vi "NewVSSNavigation.vi"() -> ()   [LabVIEW 2018]
uses:
  Vision_class/Old vision/SSL Detection Frame Simple Estimator Cameras VelCmd Folder/Core/AI Input.ctl
  Vision_class/Old vision/Controls/AI Robot.ctl
  Vision_class/Old vision/Controls/Functions Enum.ctl
  Vision_class/Old vision/Controls/AttackerStates.ctl
  Vision_class/Old vision/Controls/PathDests.ctl
  Vision_class/Old vision/Controls/PathDest.ctl
  VSSAttackerStates.ctl
  Vision_class/Old vision/SSL Detection Frame Simple Estimator Cameras VelCmd Folder/Core/AI Ball.ctl
  Vision_class/Old vision/SSL Detection Frame Simple Estimator Cameras VelCmd Folder/Core/Field Size.ctl
  Vision_class/Old vision/SSL Detection Frame Simple Estimator Cameras VelCmd Folder/Core/AI Judge.ctl
  Communication_class/Paths/MessageAI_State Folder/Intel/Command Enum.ctl
  Vision_class/Old vision/SSL Detection Frame Simple Estimator Cameras VelCmd Folder/Util/Events/Events.ctl
  Utilities_class/Utilities.lvclass
panel:
  in  "Penalty Shoot Out?":bool
  in  "PID gains Vel":T1={"proportional gain (Kc)"=0.6, "integral time (Ti, min)"=0.0, "derivative time (Td, min)"=0.0}
  in  "output angle":dbl
  in  "output xy":dbl
  in  "a1":dbl=10.0
  in  "a3":dbl=15.0
  in  "output inc":dbl
  in  "Test Mode":bool
  in  "VelNearBall":dbl=1.0 format="%#_13g"
  in  "Debug":bool
  in  "GoTo Navigation":bool
  in  "IA State Output in":T2
  out "IA State Output out":T2
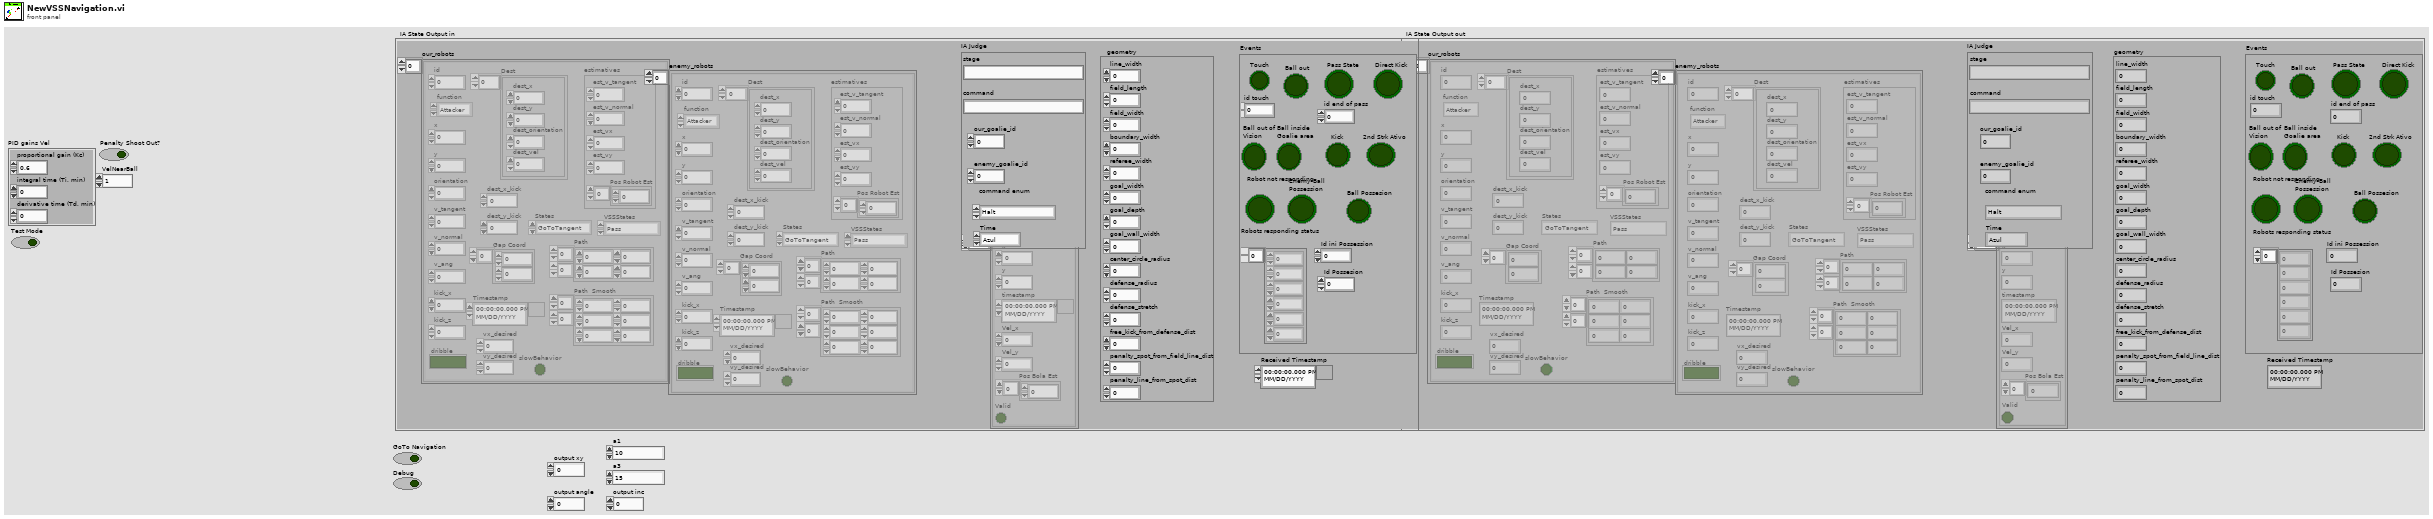
[diagram p1: front panel]
types:
  T1 = cluster{"proportional gain (Kc)":dbl, "integral time (Ti, min)":dbl, "derivative time (Td, min)":dbl}
  T2 = typedef "AI Input.ctl" = cluster{"our_robots":T3[], "enemy_robots":T3[], "balls":T9[], "geometry":T10, "IA Judge":T11, "Received Timestamp":timestamp, "Events":T13}
  T3 = typedef "AI Robot.ctl" = cluster{"id":u32, "function":T4, "x":dbl, "y":dbl, "orientation":dbl, "v_tangent":dbl, "v_normal":dbl, "v_ang":dbl, "kick_x":dbl, "kick_z":dbl, "dribble":bool, "Timestamp":timestamp, "estimatives":cluster{"est_v_tangent":dbl, "est_v_normal":dbl, "est_vx":dbl, "est_vy":dbl, "Pos Robot Est":dbl[]}, "dest_x_kick":dbl, "dest_y_kick":dbl, "Gap Coord":dbl[], "States":T5, "Path ":dbl[][], "Path  Smooth":dbl[][], "Dest":T6, "vx_desired":dbl, "vy_desired":dbl, "slowBehavior":bool, "VSSStates":T8}
  T4 = typedef "Functions Enum.ctl" = enum16{"2nd Striker", "Attacker", "Goalie", "Defender", "Striker", "Goto 0", "Dummy", "Kicker", "ZigZag 0", "ZigZag 1", "ZigZag 2", "ZigZag 3", "ZigZag 4", "ZigZag 5", "ZigZag 6", "ZigZag 7", "ZigZag 8", ""}
  T5 = typedef "AttackerStates.ctl" = enum16{"Pass", "GoToTangent", "BallGetting", "GoToKick", ""}
  T6 = typedef "PathDests.ctl" = T7[]
  T7 = typedef "PathDest.ctl" = cluster{"dest_x":dbl, "dest_y":dbl, "dest_orientation":dbl, "dest_vel":dbl}
  T8 = typedef "VSSAttackerStates.ctl" = enum16{"Pass", "GoToTangent", "BallGetting", "GoToKick", "Rotate anti-clockwise", "Rotate Clockwise", ""}
  T9 = typedef "AI Ball.ctl" = cluster{"x":dbl, "y":dbl, "timestamp":timestamp, "Vel_x":dbl, "Vel_y":dbl, "Pos Bola Est":dbl[], "Valid":bool}
  T10 = typedef "Field Size.ctl" = cluster{"line_width":u32, "field_length":u32, "field_width":u32, "boundary_width":u32, "referee_width":u32, "goal_width":u32, "goal_depth":u32, "goal_wall_width":u32, "center_circle_radius":u32, "defense_radius":u32, "defense_stretch":u32, "free_kick_from_defense_dist":u32, "penalty_spot_from_field_line_dist":u32, "penalty_line_from_spot_dist":u32}
  T11 = typedef "AI Judge.ctl" = cluster{"stage":string, "command":string, "our_goalie_id":dbl, "enemy_goalie_id":dbl, "command enum":T12, "Time":enum16{"Azul", "Amarelo"}}
  T12 = typedef "Command Enum.ctl" = enum16{"Halt", "Stop", "Force Start", "PKA Normal Start", "Prepare Kickoff Ally", "PKE Normal Start", "Prepare Kickoff Enemy", "Prepare Penalty Ally", "PPA Normal Start", "Prepare Penalty Enemy", "PPE Normal Start", "Direct Free Enemy", "Direct Free Ally", "Indirect Free Enemy", "Indirect Free Ally", "Timeout Enemy", "Timeout Ally", "Goal Enemy", "Goal Ally", "Ball Placement Enemy", "Ball Placement Ally", "Normal Half Time", "Extra Time Break", "Extra Half Time", "None", "Post Game"}
  T13 = typedef "Events.ctl" = cluster{"Touch":bool, "Ball out":bool, "id touch":dbl, "Ball out of \nVision":bool, "Ball inside \nGoalie area":bool, "Robot not responding":bool, "Robots responding status":dbl[], "Enemy Ball \nPossession":bool, "Pass State":bool, "id end of pass":dbl, "Kick":bool, "Id ini Possession":dbl, "Ball Possesion":bool, "Id Possesion":dbl, "Direct Kick":bool, "2nd Strk Ativo":bool}
  T14 = cluster{"est_v_tangent":dbl, "est_v_normal":dbl, "est_vx":dbl, "est_vy":dbl, "Pos Robot Est":dbl[]}
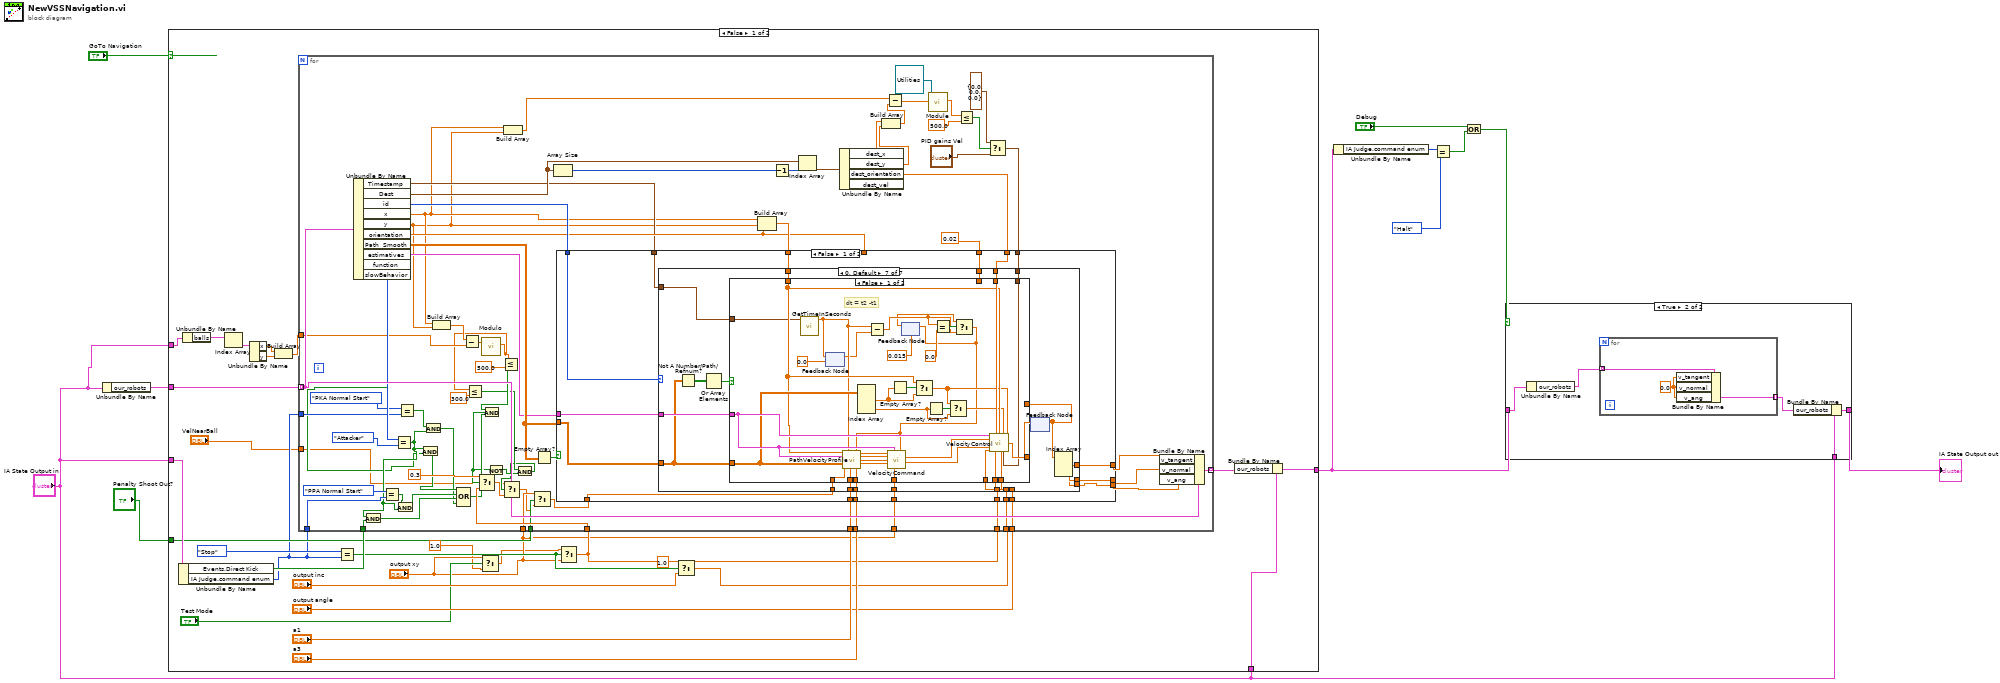
[diagram p0: block diagram]
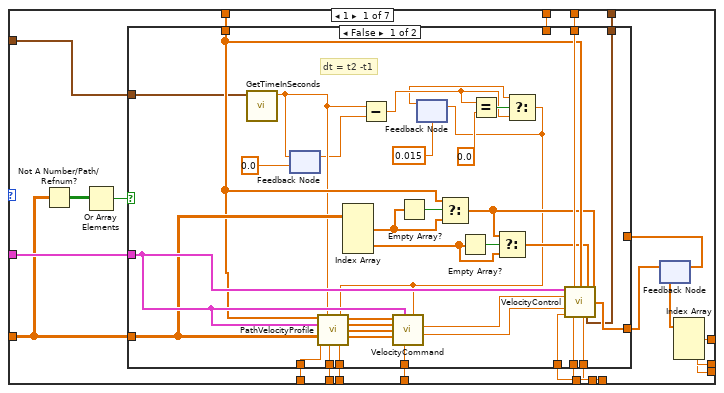
[diagram p2: hidden frame]
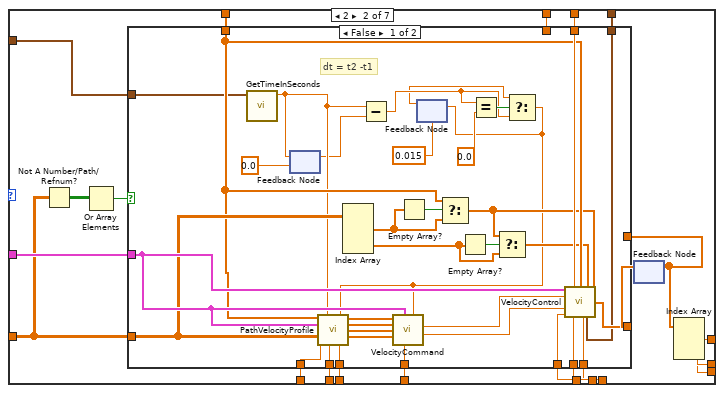
[diagram p4: hidden frame]
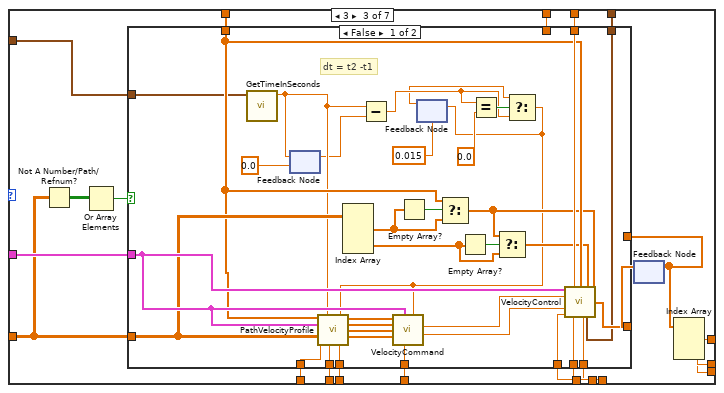
[diagram p6: hidden frame]
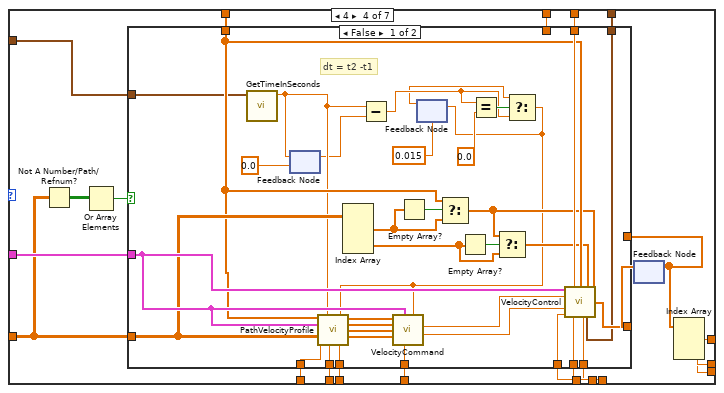
[diagram p8: hidden frame]
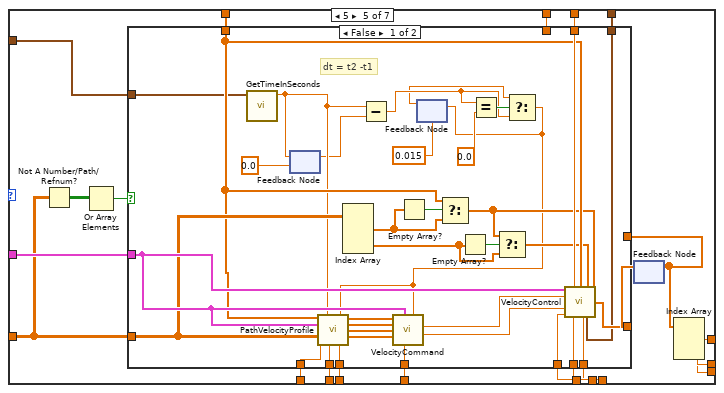
[diagram p10: hidden frame]
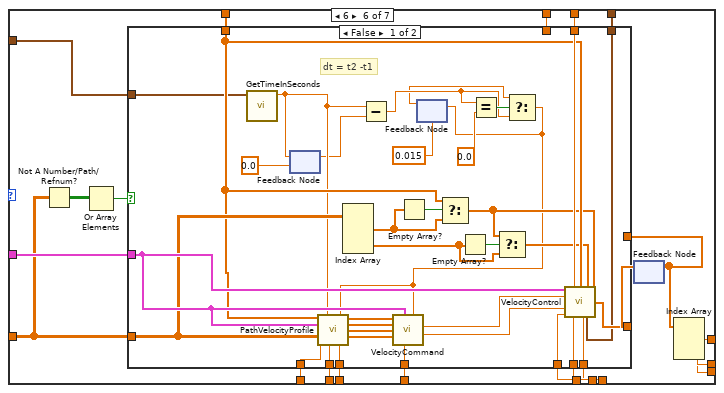
[diagram p12: hidden frame]
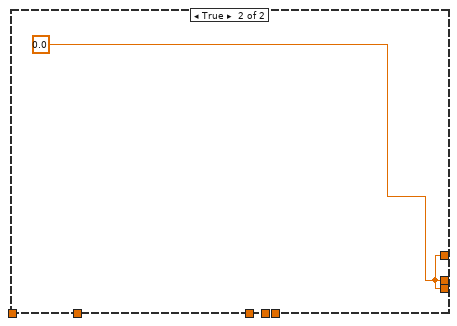
[diagram p15: hidden frame]
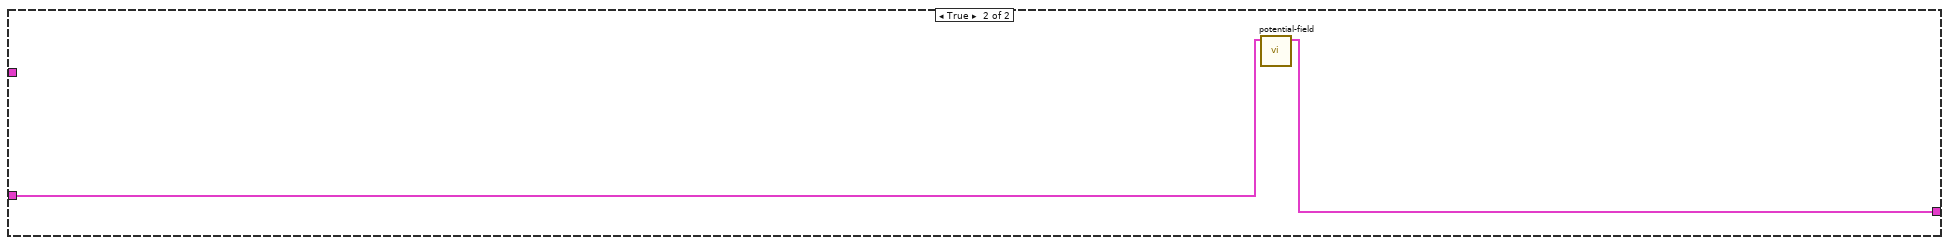
[diagram p16: hidden frame]
diagram:
  n1 = Unbundle By Name("IA State Output in") -> ("our_robots"=w11:T3[])
  n2 = case shown="False" "GoTo Navigation" {
    tunnel: w11 -> [w39 _]
    tunnel: [w36 w531] -> w8
    tunnel: "IA State Output in" -> [w32 w532]
    tunnel: "IA State Output in" -> [w37 _]
    tunnel: "IA State Output in" -> [w21 _]
    tunnel: "Penalty Shoot Out?" -> [w18 _]
    frame False {
      n3 = Unbundle By Name(w32) -> ("Events.Direct Kick"=w26:bool, "IA Judge.command enum"=w13:T12)
      n4 = Unbundle By Name(w21) -> ("balls"=w25:T9[])
      n5 = Index Array(array=w25) -> (element=w24:T9)  [unwired: 1 in]
      n6 = Unbundle By Name(w24) -> ("x"=w23:dbl, "y"=w22:dbl)
      n7 = Build Array(w23, w22) -> (w20:dbl[])
      n8 = Equal?(x=Command_Enum."Stop", y=w13) -> (x = y?=w19:bool)
      n9 = Select(t="output xy", s="Test Mode", f=1.0 ("t")) -> (s? t:f=w14:dbl)
      n10 = Select(t=w14, s=w19, f="output xy") -> (s? t:f=w30:dbl)
      n11 = Select(t=1.0, s=w19, f="output inc") -> (s? t:f=w28:dbl)
      n12 = for {
        tunnel: w39 -> [w112] mode=indexing
        tunnel: [w111] -> w38 mode=indexing
        tunnel: w30 -> [w89]
        tunnel: "a1" -> [w100]
        tunnel: "a3" -> [w99]
        tunnel: w28 -> [w95]
        tunnel: "output angle" -> [w94]
        tunnel: w30 -> [w93]
        tunnel: w13 -> [w87]
        tunnel: w26 -> [w81]
        tunnel: w13 -> [w79]
        tunnel: w20 -> [w70]
        tunnel: w18 -> [w67]
        tunnel: "output xy" -> [w66]
        tunnel: "output xy" -> [w51]
        tunnel: "VelNearBall" -> [w40]
        n13 = Unbundle By Name(w112) -> ("Timestamp"=w91:timestamp, "Dest"=w110:T6, "id"=w103:u32, "x"=w64:dbl, "y"=w63:dbl, "orientation"=w98:dbl, "Path  Smooth"=w104:dbl[][], "estimatives"=w101:T14, "function"=w80:T4, "slowBehavior"=w49:bool)
        n14 = Equal?(x=Command_Enum."PPA Normal Start", y=w87) -> (x = y?=w84:bool)
        n15 = Equal?(x=w80, y=Functions_Enum."Attacker") -> (x = y?=w76:bool)
        n16 = And(x=w76, y=w81) -> (x .and. y?=w82:bool)
        n17 = And(x=w84, y=w76) -> (x .and. y?=w83:bool)
        n18 = Equal?(x=Command_Enum."PKA Normal Start", y=w79) -> (x = y?=w77:bool)
        n19 = And(x=w76, y=w49) -> (x .and. y?=w85:bool)
        n20 = And(x=w77, y=w76) -> (x .and. y?=w75:bool)
        n21 = Build Array(w64, w63) -> (w71:dbl[])
        n22 = Compound Arithmetic op=OR(w85, w83, w82, w75) -> (w72:bool)
        n23 = Subtract(x=w71, y=w70) -> (x-y=w69:dbl[])
        n24 = call "Modulo.vi"("2D vector"=w69) -> ("Modulo"=w48:dbl)  [unwired: 10 in]
        n25 = Less Or Equal?(x=w48, y=300.0) -> (x <= y?=w46:bool)
        n26 = Less Or Equal?(x=w48, y=500.0) -> (x <= y?=w73:bool)
        n27 = And(x=w73, y=w72) -> (x .and. y?=w45:bool)
        n28 = Select(t=0.3, s=w45, f=w89) -> (s? t:f=w42:dbl)
        n29 = Not(x=w45) -> (.not. x?=w44:bool)
        n30 = Build Array(w64, w63) -> (w59:dbl[])
        n31 = And(x=w46, y=w44) -> (x .and. y?=w43:bool)
        n32 = Select(t=w40, s=w43, f=w42) -> (s? t:f=w41:dbl)
        n33 = Select(t=w66, s=w67, f=w41) -> (s? t:f=w65:dbl)
        n34 = Empty Array?(array=w104) -> (empty?=w105:bool)
        n35 = Array Size(array=w110) -> (size(s)=w109:i32)
        n36 = Build Array(w64, w63, w98) -> (w102:dbl[])
        n37 = Decrement(x=w109) -> (x-1=w108:i32)
        n38 = Index Array(array=w110, index=w108) -> (element=w107:T7)
        n39 = Unbundle By Name(w107) -> ("dest_x"=w62:dbl, "dest_y"=w61:dbl, "dest_orientation"=w106:dbl)  [unwired: 1 out]
        n40 = Build Array(w62, w61) -> (w60:dbl[])
        n41 = Subtract(x=w59, y=w60) -> (x-y=w58:dbl[])
        n42 = call-dynamic "Module.vi"("2D vector"=w58, "Utilities in"=refnum<class "Utilities.lvclass"> refnum) -> ("Modulo"=w56:dbl)  [unwired: 7 in, 2 out]
        n43 = Less Or Equal?(x=w56, y=500.0) -> (x <= y?=w54:bool)
        n44 = Select(t=T1 {"proportional gain (Kc)"=0.0, "integral time (Ti, min)"=0.0, "derivative time (Td, min)"=0.0}, s=w54, f="PID gains Vel") -> (s? t:f=w53:T1)
        n45 = case shown="False" w105 {
          tunnel: [w120 w530] -> w97
          tunnel: [w119 w530] -> w96
          tunnel: [w118 w530] -> w92
          tunnel: w103 -> [w116 _]
          tunnel: w104 -> [w122 _]
          tunnel: w106 -> [w123 _]
          tunnel: w102 -> [w121 _]
          tunnel: w101 -> [w124 _]
          tunnel: w65 -> [w130 _]
          tunnel: w100 -> [w129 _]
          tunnel: w99 -> [w128 _]
          tunnel: w98 -> [_ _]
          tunnel: w95 -> [w127 _]
          tunnel: w94 -> [w126 _]
          tunnel: w93 -> [w125 _]
          tunnel: w91 -> [w117 _]
          tunnel: 0.02 -> [w115 _]
          tunnel: w53 -> [w114 _]
          tunnel: w51 -> [w113 _]
          frame False {
            n46 = case shown="0, Default" w116 {
              tunnel: w130 -> [w151 w208 w265 w322 w379 w436 w493]
              tunnel: w129 -> [w150 w207 w264 w321 w378 w435 w492]
              tunnel: w128 -> [w149 w206 w263 w320 w377 w434 w491]
              tunnel: w127 -> [w148 w205 w262 w319 w376 w433 w490]
              tunnel: w126 -> [w147 w204 w261 w318 w375 w432 w489]
              tunnel: w125 -> [w146 w203 w260 w317 w374 w431 w488]
              tunnel: w124 -> [w145 w202 w259 w316 w373 w430 w487]
              tunnel: w123 -> [w144 w201 w258 w315 w372 w429 w486]
              tunnel: w122 -> [w136 w193 w250 w307 w364 w421 w478]
              tunnel: w121 -> [w143 w200 w257 w314 w371 w428 w485]
              tunnel: [w142 w199 w256 w313 w370 w427 w484] -> w120
              tunnel: [w141 w198 w255 w312 w369 w426 w483] -> w119
              tunnel: [w140 w197 w254 w311 w368 w425 w482] -> w118
              tunnel: w117 -> [w139 w196 w253 w310 w367 w424 w481]
              tunnel: w115 -> [w133 w190 w247 w304 w361 w418 w475]
              tunnel: w114 -> [w132 w189 w246 w303 w360 w417 w474]
              tunnel: w113 -> [w131 w188 w245 w302 w359 w416 w473]
              frame 1 {
                n47 = Not A Number/Path/Refnum?(number/path/refnum=w136) -> (NaN/Path/Refnum?=w135:bool[][])
                n48 = Or Array Elements(Boolean array=w135) -> (logical OR=w134:bool)
                n49 = feedback #1() -> (w137:dbl[])  [unwired: 1 in]
                n50 = case shown="False" w134 {
                  tunnel: w151 -> [w186 _]
                  tunnel: w150 -> [w185 _]
                  tunnel: w149 -> [w184 _]
                  tunnel: w148 -> [w183 _]
                  tunnel: w147 -> [w182 _]
                  tunnel: w146 -> [w181 _]
                  tunnel: w145 -> [w180 _]
                  tunnel: w144 -> [w179 _]
                  tunnel: w136 -> [w178 _]
                  tunnel: w143 -> [w177 _]
                  tunnel: [w176 w187] -> w138
                  tunnel: w139 -> [w163 _]
                  tunnel: w137 -> [_ w187]
                  tunnel: w133 -> [_ _]
                  tunnel: w132 -> [w154 _]
                  tunnel: w131 -> [w152 _]
                  frame False {
                    # "dt = t2 -t1"
                    n51 = call "GetTimeInSeconds.vi"("Timestamp"=w163) -> ("Numeric"=w157:dbl)  [unwired: 10 in]
                    n52 = feedback-in #2(w157) -> ()
                    n53 = feedback #2(0.0 ("Numeric")) -> (w156:dbl)
                    n54 = Index Array(array=w178) -> (element #1=w165:dbl[], element #2=w168:dbl[])  [unwired: 4 in]
                    n55 = Subtract(x=w157, y=w156) -> (x-y=w159:dbl)
                    n56 = Empty Array?(array=w165) -> (empty?=w166:bool)
                    n57 = feedback #3(0.015 ("Numeric")) -> (w158:dbl)
                    n58 = Select(t=w177, s=w166, f=w165) -> (s? t:f=w164:dbl[])
                    n59 = Empty Array?(array=w168) -> (empty?=w169:bool)
                    n60 = Equal?(x=w159, y=0.0) -> (x = y?=w162:bool)
                    n61 = Select(t=w164, s=w169, f=w168) -> (s? t:f=w167:dbl[])
                    n62 = Select(t=w158, s=w162, f=w159) -> (s? t:f=w153:dbl)
                    n63 = call "PathVelocityProfile.vi"("Pose"=w177, "time"=w157, "intervalo"=w153, "estimatives"=w180, "Path  Smooth"=w178, "V_max"=w186, "Accel"=w185, "DesAccel"=w184) -> ("Time X"=w175:dbl[], "Velocities X"=w174:dbl[], "Time Y"=w173:dbl[], "Velocities Y"=w172:dbl[])  [unwired: 4 in]
                    n64 = call "VelocityCommand.vi"("intervalo"=w153, "MaxOutputXY"=w152, "estimatives"=w180, "Velocities Y"=w172, "Time Y"=w173, "Velocities X"=w174, "Time X"=w175) -> ("Vy"=w171:dbl, "Vx"=w170:dbl)  [unwired: 3 in]
                    n65 = feedback-in #3(w153) -> ()
                    n66 = call "VelocityControl.vi"("estimatives"=w180, "Dest_orientation"=w179, "Position"=w177, "Waypoint 1"=w167, "Waypoint 0"=w164, "Vx"=w170, "Vy"=w171, "output xy"=w181, "output inc"=w183, "output angle"=w182, "PID gains Vel"=w154) -> ("Output Velocity"=w176:dbl[])  [unwired: 4 in]
                  }
                  frame True {
                  }
                }
                n67 = feedback-in #1(w138) -> ()
                n68 = Index Array(array=w137) -> (element #1=w142:dbl, element #2=w141:dbl, element #3=w140:dbl)  [unwired: 3 in]
              }
              frame 2 {
                n69 = Not A Number/Path/Refnum?(number/path/refnum=w193) -> (NaN/Path/Refnum?=w192:bool[][])
                n70 = Or Array Elements(Boolean array=w192) -> (logical OR=w191:bool)
                n71 = feedback #4() -> (w194:dbl[])  [unwired: 1 in]
                n72 = case shown="False" w191 {
                  tunnel: w208 -> [w243 _]
                  tunnel: w207 -> [w242 _]
                  tunnel: w206 -> [w241 _]
                  tunnel: w205 -> [w240 _]
                  tunnel: w204 -> [w239 _]
                  tunnel: w203 -> [w238 _]
                  tunnel: w202 -> [w237 _]
                  tunnel: w201 -> [w236 _]
                  tunnel: w193 -> [w235 _]
                  tunnel: w200 -> [w234 _]
                  tunnel: [w233 w244] -> w195
                  tunnel: w196 -> [w220 _]
                  tunnel: w194 -> [_ w244]
                  tunnel: w190 -> [_ _]
                  tunnel: w189 -> [w211 _]
                  tunnel: w188 -> [w209 _]
                  frame False {
                    # "dt = t2 -t1"
                    n73 = call "GetTimeInSeconds.vi"("Timestamp"=w220) -> ("Numeric"=w214:dbl)  [unwired: 10 in]
                    n74 = feedback-in #5(w214) -> ()
                    n75 = feedback #5(0.0 ("Numeric")) -> (w213:dbl)
                    n76 = Index Array(array=w235) -> (element #1=w222:dbl[], element #2=w225:dbl[])  [unwired: 4 in]
                    n77 = Subtract(x=w214, y=w213) -> (x-y=w216:dbl)
                    n78 = Empty Array?(array=w222) -> (empty?=w223:bool)
                    n79 = feedback #6(0.015 ("Numeric")) -> (w215:dbl)
                    n80 = Select(t=w234, s=w223, f=w222) -> (s? t:f=w221:dbl[])
                    n81 = Empty Array?(array=w225) -> (empty?=w226:bool)
                    n82 = Equal?(x=w216, y=0.0) -> (x = y?=w219:bool)
                    n83 = Select(t=w221, s=w226, f=w225) -> (s? t:f=w224:dbl[])
                    n84 = Select(t=w215, s=w219, f=w216) -> (s? t:f=w210:dbl)
                    n85 = call "PathVelocityProfile.vi"("Pose"=w234, "time"=w214, "intervalo"=w210, "estimatives"=w237, "Path  Smooth"=w235, "V_max"=w243, "Accel"=w242, "DesAccel"=w241) -> ("Time X"=w232:dbl[], "Velocities X"=w231:dbl[], "Time Y"=w230:dbl[], "Velocities Y"=w229:dbl[])  [unwired: 4 in]
                    n86 = call "VelocityCommand.vi"("intervalo"=w210, "MaxOutputXY"=w209, "estimatives"=w237, "Velocities Y"=w229, "Time Y"=w230, "Velocities X"=w231, "Time X"=w232) -> ("Vy"=w228:dbl, "Vx"=w227:dbl)  [unwired: 3 in]
                    n87 = feedback-in #6(w210) -> ()
                    n88 = call "VelocityControl.vi"("estimatives"=w237, "Dest_orientation"=w236, "Position"=w234, "Waypoint 1"=w224, "Waypoint 0"=w221, "Vx"=w227, "Vy"=w228, "output xy"=w238, "output inc"=w240, "output angle"=w239, "PID gains Vel"=w211) -> ("Output Velocity"=w233:dbl[])  [unwired: 4 in]
                  }
                  frame True {
                  }
                }
                n89 = feedback-in #4(w195) -> ()
                n90 = Index Array(array=w194) -> (element #1=w199:dbl, element #2=w198:dbl, element #3=w197:dbl)  [unwired: 3 in]
              }
              frame 3 {
                n91 = Not A Number/Path/Refnum?(number/path/refnum=w250) -> (NaN/Path/Refnum?=w249:bool[][])
                n92 = Or Array Elements(Boolean array=w249) -> (logical OR=w248:bool)
                n93 = feedback #7() -> (w251:dbl[])  [unwired: 1 in]
                n94 = case shown="False" w248 {
                  tunnel: w265 -> [w300 _]
                  tunnel: w264 -> [w299 _]
                  tunnel: w263 -> [w298 _]
                  tunnel: w262 -> [w297 _]
                  tunnel: w261 -> [w296 _]
                  tunnel: w260 -> [w295 _]
                  tunnel: w259 -> [w294 _]
                  tunnel: w258 -> [w293 _]
                  tunnel: w250 -> [w292 _]
                  tunnel: w257 -> [w291 _]
                  tunnel: [w290 w301] -> w252
                  tunnel: w253 -> [w277 _]
                  tunnel: w251 -> [_ w301]
                  tunnel: w247 -> [_ _]
                  tunnel: w246 -> [w268 _]
                  tunnel: w245 -> [w266 _]
                  frame False {
                    # "dt = t2 -t1"
                    n95 = call "GetTimeInSeconds.vi"("Timestamp"=w277) -> ("Numeric"=w271:dbl)  [unwired: 10 in]
                    n96 = feedback-in #8(w271) -> ()
                    n97 = feedback #8(0.0 ("Numeric")) -> (w270:dbl)
                    n98 = Index Array(array=w292) -> (element #1=w279:dbl[], element #2=w282:dbl[])  [unwired: 4 in]
                    n99 = Subtract(x=w271, y=w270) -> (x-y=w273:dbl)
                    n100 = Empty Array?(array=w279) -> (empty?=w280:bool)
                    n101 = feedback #9(0.015 ("Numeric")) -> (w272:dbl)
                    n102 = Select(t=w291, s=w280, f=w279) -> (s? t:f=w278:dbl[])
                    n103 = Empty Array?(array=w282) -> (empty?=w283:bool)
                    n104 = Equal?(x=w273, y=0.0) -> (x = y?=w276:bool)
                    n105 = Select(t=w278, s=w283, f=w282) -> (s? t:f=w281:dbl[])
                    n106 = Select(t=w272, s=w276, f=w273) -> (s? t:f=w267:dbl)
                    n107 = call "PathVelocityProfile.vi"("Pose"=w291, "time"=w271, "intervalo"=w267, "estimatives"=w294, "Path  Smooth"=w292, "V_max"=w300, "Accel"=w299, "DesAccel"=w298) -> ("Time X"=w289:dbl[], "Velocities X"=w288:dbl[], "Time Y"=w287:dbl[], "Velocities Y"=w286:dbl[])  [unwired: 4 in]
                    n108 = call "VelocityCommand.vi"("intervalo"=w267, "MaxOutputXY"=w266, "estimatives"=w294, "Velocities Y"=w286, "Time Y"=w287, "Velocities X"=w288, "Time X"=w289) -> ("Vy"=w285:dbl, "Vx"=w284:dbl)  [unwired: 3 in]
                    n109 = feedback-in #9(w267) -> ()
                    n110 = call "VelocityControl.vi"("estimatives"=w294, "Dest_orientation"=w293, "Position"=w291, "Waypoint 1"=w281, "Waypoint 0"=w278, "Vx"=w284, "Vy"=w285, "output xy"=w295, "output inc"=w297, "output angle"=w296, "PID gains Vel"=w268) -> ("Output Velocity"=w290:dbl[])  [unwired: 4 in]
                  }
                  frame True {
                  }
                }
                n111 = feedback-in #7(w252) -> ()
                n112 = Index Array(array=w251) -> (element #1=w256:dbl, element #2=w255:dbl, element #3=w254:dbl)  [unwired: 3 in]
              }
              frame 4 {
                n113 = Not A Number/Path/Refnum?(number/path/refnum=w307) -> (NaN/Path/Refnum?=w306:bool[][])
                n114 = Or Array Elements(Boolean array=w306) -> (logical OR=w305:bool)
                n115 = feedback #10() -> (w308:dbl[])  [unwired: 1 in]
                n116 = case shown="False" w305 {
                  tunnel: w322 -> [w357 _]
                  tunnel: w321 -> [w356 _]
                  tunnel: w320 -> [w355 _]
                  tunnel: w319 -> [w354 _]
                  tunnel: w318 -> [w353 _]
                  tunnel: w317 -> [w352 _]
                  tunnel: w316 -> [w351 _]
                  tunnel: w315 -> [w350 _]
                  tunnel: w307 -> [w349 _]
                  tunnel: w314 -> [w348 _]
                  tunnel: [w347 w358] -> w309
                  tunnel: w310 -> [w334 _]
                  tunnel: w308 -> [_ w358]
                  tunnel: w304 -> [_ _]
                  tunnel: w303 -> [w325 _]
                  tunnel: w302 -> [w323 _]
                  frame False {
                    # "dt = t2 -t1"
                    n117 = call "GetTimeInSeconds.vi"("Timestamp"=w334) -> ("Numeric"=w328:dbl)  [unwired: 10 in]
                    n118 = feedback-in #11(w328) -> ()
                    n119 = feedback #11(0.0 ("Numeric")) -> (w327:dbl)
                    n120 = Index Array(array=w349) -> (element #1=w336:dbl[], element #2=w339:dbl[])  [unwired: 4 in]
                    n121 = Subtract(x=w328, y=w327) -> (x-y=w330:dbl)
                    n122 = Empty Array?(array=w336) -> (empty?=w337:bool)
                    n123 = feedback #12(0.015 ("Numeric")) -> (w329:dbl)
                    n124 = Select(t=w348, s=w337, f=w336) -> (s? t:f=w335:dbl[])
                    n125 = Empty Array?(array=w339) -> (empty?=w340:bool)
                    n126 = Equal?(x=w330, y=0.0) -> (x = y?=w333:bool)
                    n127 = Select(t=w335, s=w340, f=w339) -> (s? t:f=w338:dbl[])
                    n128 = Select(t=w329, s=w333, f=w330) -> (s? t:f=w324:dbl)
                    n129 = call "PathVelocityProfile.vi"("Pose"=w348, "time"=w328, "intervalo"=w324, "estimatives"=w351, "Path  Smooth"=w349, "V_max"=w357, "Accel"=w356, "DesAccel"=w355) -> ("Time X"=w346:dbl[], "Velocities X"=w345:dbl[], "Time Y"=w344:dbl[], "Velocities Y"=w343:dbl[])  [unwired: 4 in]
                    n130 = call "VelocityCommand.vi"("intervalo"=w324, "MaxOutputXY"=w323, "estimatives"=w351, "Velocities Y"=w343, "Time Y"=w344, "Velocities X"=w345, "Time X"=w346) -> ("Vy"=w342:dbl, "Vx"=w341:dbl)  [unwired: 3 in]
                    n131 = feedback-in #12(w324) -> ()
                    n132 = call "VelocityControl.vi"("estimatives"=w351, "Dest_orientation"=w350, "Position"=w348, "Waypoint 1"=w338, "Waypoint 0"=w335, "Vx"=w341, "Vy"=w342, "output xy"=w352, "output inc"=w354, "output angle"=w353, "PID gains Vel"=w325) -> ("Output Velocity"=w347:dbl[])  [unwired: 4 in]
                  }
                  frame True {
                  }
                }
                n133 = feedback-in #10(w309) -> ()
                n134 = Index Array(array=w308) -> (element #1=w313:dbl, element #2=w312:dbl, element #3=w311:dbl)  [unwired: 3 in]
              }
              frame 5 {
                n135 = Not A Number/Path/Refnum?(number/path/refnum=w364) -> (NaN/Path/Refnum?=w363:bool[][])
                n136 = Or Array Elements(Boolean array=w363) -> (logical OR=w362:bool)
                n137 = feedback #13() -> (w365:dbl[])  [unwired: 1 in]
                n138 = case shown="False" w362 {
                  tunnel: w379 -> [w414 _]
                  tunnel: w378 -> [w413 _]
                  tunnel: w377 -> [w412 _]
                  tunnel: w376 -> [w411 _]
                  tunnel: w375 -> [w410 _]
                  tunnel: w374 -> [w409 _]
                  tunnel: w373 -> [w408 _]
                  tunnel: w372 -> [w407 _]
                  tunnel: w364 -> [w406 _]
                  tunnel: w371 -> [w405 _]
                  tunnel: [w404 w415] -> w366
                  tunnel: w367 -> [w391 _]
                  tunnel: w365 -> [_ w415]
                  tunnel: w361 -> [_ _]
                  tunnel: w360 -> [w382 _]
                  tunnel: w359 -> [w380 _]
                  frame False {
                    # "dt = t2 -t1"
                    n139 = call "GetTimeInSeconds.vi"("Timestamp"=w391) -> ("Numeric"=w385:dbl)  [unwired: 10 in]
                    n140 = feedback-in #14(w385) -> ()
                    n141 = feedback #14(0.0 ("Numeric")) -> (w384:dbl)
                    n142 = Index Array(array=w406) -> (element #1=w393:dbl[], element #2=w396:dbl[])  [unwired: 4 in]
                    n143 = Subtract(x=w385, y=w384) -> (x-y=w387:dbl)
                    n144 = Empty Array?(array=w393) -> (empty?=w394:bool)
                    n145 = feedback #15(0.015 ("Numeric")) -> (w386:dbl)
                    n146 = Select(t=w405, s=w394, f=w393) -> (s? t:f=w392:dbl[])
                    n147 = Empty Array?(array=w396) -> (empty?=w397:bool)
                    n148 = Equal?(x=w387, y=0.0) -> (x = y?=w390:bool)
                    n149 = Select(t=w392, s=w397, f=w396) -> (s? t:f=w395:dbl[])
                    n150 = Select(t=w386, s=w390, f=w387) -> (s? t:f=w381:dbl)
                    n151 = call "PathVelocityProfile.vi"("Pose"=w405, "time"=w385, "intervalo"=w381, "estimatives"=w408, "Path  Smooth"=w406, "V_max"=w414, "Accel"=w413, "DesAccel"=w412) -> ("Time X"=w403:dbl[], "Velocities X"=w402:dbl[], "Time Y"=w401:dbl[], "Velocities Y"=w400:dbl[])  [unwired: 4 in]
                    n152 = call "VelocityCommand.vi"("intervalo"=w381, "MaxOutputXY"=w380, "estimatives"=w408, "Velocities Y"=w400, "Time Y"=w401, "Velocities X"=w402, "Time X"=w403) -> ("Vy"=w399:dbl, "Vx"=w398:dbl)  [unwired: 3 in]
                    n153 = feedback-in #15(w381) -> ()
                    n154 = call "VelocityControl.vi"("estimatives"=w408, "Dest_orientation"=w407, "Position"=w405, "Waypoint 1"=w395, "Waypoint 0"=w392, "Vx"=w398, "Vy"=w399, "output xy"=w409, "output inc"=w411, "output angle"=w410, "PID gains Vel"=w382) -> ("Output Velocity"=w404:dbl[])  [unwired: 4 in]
                  }
                  frame True {
                  }
                }
                n155 = feedback-in #13(w366) -> ()
                n156 = Index Array(array=w365) -> (element #1=w370:dbl, element #2=w369:dbl, element #3=w368:dbl)  [unwired: 3 in]
              }
              frame 6 {
                n157 = Not A Number/Path/Refnum?(number/path/refnum=w421) -> (NaN/Path/Refnum?=w420:bool[][])
                n158 = Or Array Elements(Boolean array=w420) -> (logical OR=w419:bool)
                n159 = feedback #16() -> (w422:dbl[])  [unwired: 1 in]
                n160 = case shown="False" w419 {
                  tunnel: w436 -> [w471 _]
                  tunnel: w435 -> [w470 _]
                  tunnel: w434 -> [w469 _]
                  tunnel: w433 -> [w468 _]
                  tunnel: w432 -> [w467 _]
                  tunnel: w431 -> [w466 _]
                  tunnel: w430 -> [w465 _]
                  tunnel: w429 -> [w464 _]
                  tunnel: w421 -> [w463 _]
                  tunnel: w428 -> [w462 _]
                  tunnel: [w461 w472] -> w423
                  tunnel: w424 -> [w448 _]
                  tunnel: w422 -> [_ w472]
                  tunnel: w418 -> [_ _]
                  tunnel: w417 -> [w439 _]
                  tunnel: w416 -> [w437 _]
                  frame False {
                    # "dt = t2 -t1"
                    n161 = call "GetTimeInSeconds.vi"("Timestamp"=w448) -> ("Numeric"=w442:dbl)  [unwired: 10 in]
                    n162 = feedback-in #17(w442) -> ()
                    n163 = feedback #17(0.0 ("Numeric")) -> (w441:dbl)
                    n164 = Index Array(array=w463) -> (element #1=w450:dbl[], element #2=w453:dbl[])  [unwired: 4 in]
                    n165 = Subtract(x=w442, y=w441) -> (x-y=w444:dbl)
                    n166 = Empty Array?(array=w450) -> (empty?=w451:bool)
                    n167 = feedback #18(0.015 ("Numeric")) -> (w443:dbl)
                    n168 = Select(t=w462, s=w451, f=w450) -> (s? t:f=w449:dbl[])
                    n169 = Empty Array?(array=w453) -> (empty?=w454:bool)
                    n170 = Equal?(x=w444, y=0.0) -> (x = y?=w447:bool)
                    n171 = Select(t=w449, s=w454, f=w453) -> (s? t:f=w452:dbl[])
                    n172 = Select(t=w443, s=w447, f=w444) -> (s? t:f=w438:dbl)
                    n173 = call "PathVelocityProfile.vi"("Pose"=w462, "time"=w442, "intervalo"=w438, "estimatives"=w465, "Path  Smooth"=w463, "V_max"=w471, "Accel"=w470, "DesAccel"=w469) -> ("Time X"=w460:dbl[], "Velocities X"=w459:dbl[], "Time Y"=w458:dbl[], "Velocities Y"=w457:dbl[])  [unwired: 4 in]
                    n174 = call "VelocityCommand.vi"("intervalo"=w438, "MaxOutputXY"=w437, "estimatives"=w465, "Velocities Y"=w457, "Time Y"=w458, "Velocities X"=w459, "Time X"=w460) -> ("Vy"=w456:dbl, "Vx"=w455:dbl)  [unwired: 3 in]
                    n175 = feedback-in #18(w438) -> ()
                    n176 = call "VelocityControl.vi"("estimatives"=w465, "Dest_orientation"=w464, "Position"=w462, "Waypoint 1"=w452, "Waypoint 0"=w449, "Vx"=w455, "Vy"=w456, "output xy"=w466, "output inc"=w468, "output angle"=w467, "PID gains Vel"=w439) -> ("Output Velocity"=w461:dbl[])  [unwired: 4 in]
                  }
                  frame True {
                  }
                }
                n177 = feedback-in #16(w423) -> ()
                n178 = Index Array(array=w422) -> (element #1=w427:dbl, element #2=w426:dbl, element #3=w425:dbl)  [unwired: 3 in]
              }
              frame 0, Default {
                n179 = Not A Number/Path/Refnum?(number/path/refnum=w478) -> (NaN/Path/Refnum?=w477:bool[][])
                n180 = Or Array Elements(Boolean array=w477) -> (logical OR=w476:bool)
                n181 = feedback #19() -> (w479:dbl[])  [unwired: 1 in]
                n182 = case shown="False" w476 {
                  tunnel: w493 -> [w528 _]
                  tunnel: w492 -> [w527 _]
                  tunnel: w491 -> [w526 _]
                  tunnel: w490 -> [w525 _]
                  tunnel: w489 -> [w524 _]
                  tunnel: w488 -> [w523 _]
                  tunnel: w487 -> [w522 _]
                  tunnel: w486 -> [w521 _]
                  tunnel: w478 -> [w520 _]
                  tunnel: w485 -> [w519 _]
                  tunnel: [w518 w529] -> w480
                  tunnel: w481 -> [w505 _]
                  tunnel: w479 -> [_ w529]
                  tunnel: w475 -> [_ _]
                  tunnel: w474 -> [w496 _]
                  tunnel: w473 -> [w494 _]
                  frame False {
                    # "dt = t2 -t1"
                    n183 = call "GetTimeInSeconds.vi"("Timestamp"=w505) -> ("Numeric"=w499:dbl)  [unwired: 10 in]
                    n184 = feedback-in #20(w499) -> ()
                    n185 = feedback #20(0.0 ("Numeric")) -> (w498:dbl)
                    n186 = Index Array(array=w520) -> (element #1=w507:dbl[], element #2=w510:dbl[])  [unwired: 4 in]
                    n187 = Subtract(x=w499, y=w498) -> (x-y=w501:dbl)
                    n188 = Empty Array?(array=w507) -> (empty?=w508:bool)
                    n189 = feedback #21(0.015 ("Numeric")) -> (w500:dbl)
                    n190 = Select(t=w519, s=w508, f=w507) -> (s? t:f=w506:dbl[])
                    n191 = Empty Array?(array=w510) -> (empty?=w511:bool)
                    n192 = Equal?(x=w501, y=0.0) -> (x = y?=w504:bool)
                    n193 = Select(t=w506, s=w511, f=w510) -> (s? t:f=w509:dbl[])
                    n194 = Select(t=w500, s=w504, f=w501) -> (s? t:f=w495:dbl)
                    n195 = call "PathVelocityProfile.vi"("Pose"=w519, "time"=w499, "intervalo"=w495, "estimatives"=w522, "Path  Smooth"=w520, "V_max"=w528, "Accel"=w527, "DesAccel"=w526) -> ("Time X"=w517:dbl[], "Velocities X"=w516:dbl[], "Time Y"=w515:dbl[], "Velocities Y"=w514:dbl[])  [unwired: 4 in]
                    n196 = call "VelocityCommand.vi"("intervalo"=w495, "MaxOutputXY"=w494, "estimatives"=w522, "Velocities Y"=w514, "Time Y"=w515, "Velocities X"=w516, "Time X"=w517) -> ("Vy"=w513:dbl, "Vx"=w512:dbl)  [unwired: 3 in]
                    n197 = feedback-in #21(w495) -> ()
                    n198 = call "VelocityControl.vi"("estimatives"=w522, "Dest_orientation"=w521, "Position"=w519, "Waypoint 1"=w509, "Waypoint 0"=w506, "Vx"=w512, "Vy"=w513, "output xy"=w523, "output inc"=w525, "output angle"=w524, "PID gains Vel"=w496) -> ("Output Velocity"=w518:dbl[])  [unwired: 4 in]
                  }
                  frame True {
                  }
                }
                n199 = feedback-in #19(w480) -> ()
                n200 = Index Array(array=w479) -> (element #1=w484:dbl, element #2=w483:dbl, element #3=w482:dbl)  [unwired: 3 in]
              }
            }
          }
          frame True {
            w530 = 0.0 ("output")
          }
        }
        n201 = Bundle By Name(cluster=w112, "v_tangent"=w97, "v_normal"=w96, "v_ang"=w92) -> (w111:T3)
      }
      n202 = Bundle By Name(cluster=w37, "our_robots"=w38) -> (w36:T2)
    }
    frame True {
      n203 = call "potential-field.vi"("IA State Output in"=w532) -> ("IA State Output out"=w531:T2)  [unwired: 10 in]
    }
  }
  n204 = Unbundle By Name(w8) -> ("IA Judge.command enum"=w7:T12)
  n205 = Equal?(x=w7, y=Command_Enum."Halt") -> (x = y?=w4:bool)
  n206 = Or(x="Debug", y=w4) -> (x .or. y?=w5:bool)
  n207 = case shown="True" w5 {
    tunnel: [w533 w538] -> w9
    tunnel: w8 -> [w533 w535]
    tunnel: "IA State Output in" -> [_ w536]
    frame False {
    }
    frame True {
      n208 = Unbundle By Name(w535) -> ("our_robots"=w534:T3[])
      n209 = for {
        tunnel: [w541] -> w537 mode=indexing
        tunnel: w534 -> [w539] mode=indexing
        w540 = 0.0 ("v_normal")
        n210 = Bundle By Name(cluster=w539, "v_tangent"=w540, "v_normal"=w540, "v_ang"=w540) -> (w541:T3)
      }
      n211 = Bundle By Name(cluster=w536, "our_robots"=w537) -> (w538:T2)
    }
  }
  "IA State Output out" <- w9
